vi "Test Harness.vi"() -> ()   [LabVIEW 2018]
panel:
  in  "Server Closed":string="The server VI closed the connection."
  in  "Stop":bool
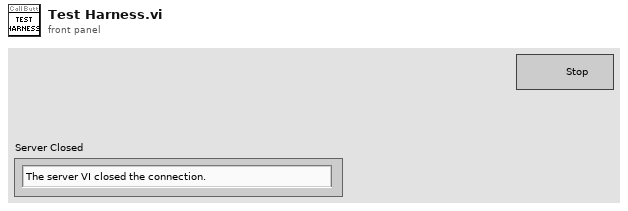
[diagram p1: front panel]
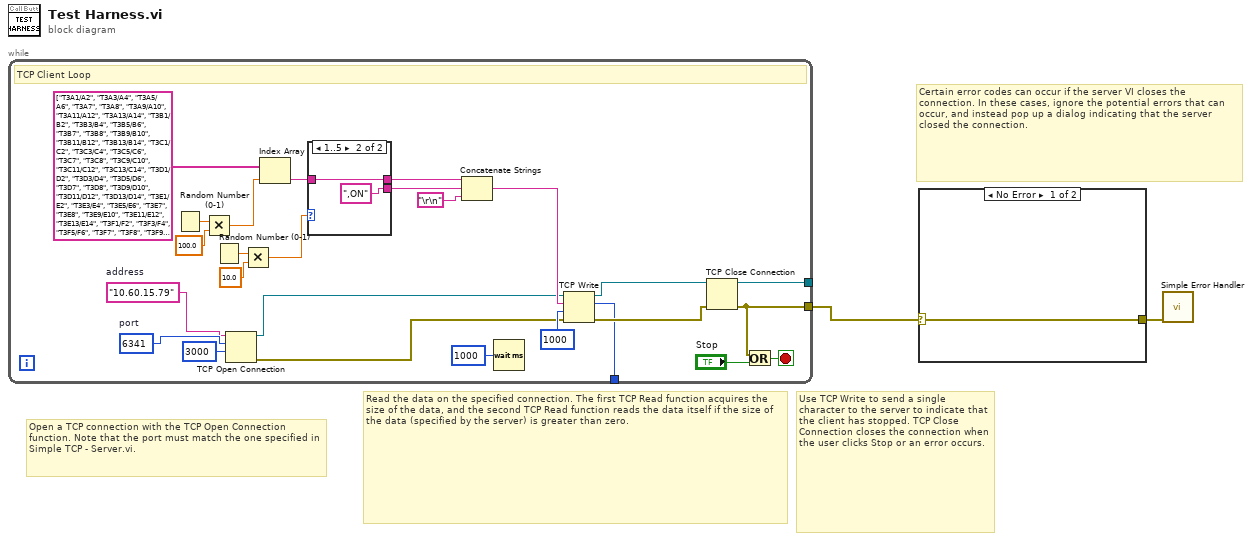
[diagram p0: block diagram]
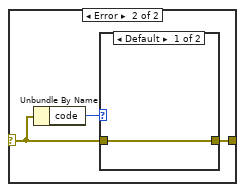
[diagram p2: hidden frame]
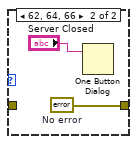
[diagram p3: hidden frame]
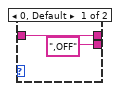
[diagram p4: hidden frame]
diagram:
  # "Certain error codes can occur if the server VI closes the connection. In these cases, ignore the potential errors that can occur, and instead pop up a dialog indicating that the server closed the connection."
  # "Use TCP Write to send a single character to the server to indicate that the client has stopped. TCP Close Connection closes the connection when the user clicks Stop or an error occurs."
  # "Read the data on the specified connection. The first TCP Read function acquires the size of the data, and the second TCP Read function reads the data itself if the size of the data (specified by the server) is greater than zero."
  # "Open a TCP connection with the TCP Open Connection function. Note that the port must match the one specified in Simple TCP - Server.vi."
  n1 = while {
    tunnel: [w10] -> w1
    tunnel: [w9] -> _
    tunnel: [w3] -> _
    stop <- w27 stop-if-true
    w7 = u16 6341  # port
    w6 = "10.60.15.79"  # address
    # "TCP Client Loop"
    n2 = Random Number (0-1)() -> (number: 0 to 1=w23:dbl)
    n3 = Multiply(x=w23, y=100.0) -> (x*y=w21:dbl)
    n4 = Random Number (0-1)() -> (number: 0 to 1=w15:dbl)
    n5 = TCP Open Connection(address=w6, remote port or service name=w7, timeout ms (60000)=3000) -> (connection ID=w5:refnum<k5>, error out=w4:errorcluster)  [unwired: 2 in]
    n6 = Multiply(x=w15, y=10.0) -> (x*y=w14:dbl)
    n7 = Index Array(array=string[] ["T3A1/A2", "T3A3/A4", "T3A5/A6", "T3A7", "T3A8", "T3A9/A10", "T3A11/A12", "T3A13/A14", "T3B1/B2", "T3B3/B4", "T3B5/B6", "T3B7", "T3B8", "T3B9/B10", "T3B11/B12", "T3B13/B14", "T3C1/C2", "T3C3/C4", "T3C5/C6", "T3C7", "T3C8", "T3C9/C10", "T3C11/C12", "T3C13/C14", "T3D1/D2", "T3D3/D4", "T3D5/D6", "T3D7", "T3D8", "T3D9/D10", "T3D11/D12", "T3D13/D14", "T3E1/E2", "T3E3/E4", "T3E5/E6", "T3E7", "T3E8", "T3E9/E10", "T3E11/E12", "T3E13/E14", "T3F1/F2", "T3F3/F4", "T3F5/F6", "T3F7", "T3F8", "T3F9/F10", "T3F11/F12", "T3F13/F14", "T3G1/G2", "T3G3/G4", "T3G5/G6", "T3G7", "T3G8", "T3G9/G10", "T3G11/G12", "T3G13/G14", "T3H1/H2", "T3H3/H4", "T3H5", "I1", "I2", "I3", "Quit", "T2B1/B2", "T2B3/B4", "T2B5/B6", "T2B7", "T2B8", "T2B9/B10", "T2B11/B12", "T2B13/B14", "T2C1/C2", "T2C3/C4", "T2C5/C6", "T2C7", "T2C8", "T2C9/C10", "T2C11/C12", "T2C13/C14", "T2D1/D2", "T2D3/D4", "T2D5/D6", "T2D7", "T2D8", "T2D9/D10", "T2D11/D12", "T2D13/D14", "T2E3/E4", "T2E5/E6", "T2E7", "T2E8", "T2E9/E10", "T2E11/E12", "T2E13/E14", "T2F1/F2", "T2F3", "T2F4/F5", "T2F6/F7", "T2G1/G2", "T2G3/G4", "T2A3/A4", "T2A5/A6", "T2A7", "T2A8", "T2A9/A10", "T2A11/A12", "T2A13/A13", "T2A1/A2", "T1B1/B2", "T1B3/B4", "T1B5/B6", "T1B7", "T1B8", "T1B9/B10", "T1B11/B12", "T1B13/B14", "T1C1/C2", "T1C3/C4", "T1C5/C6", "T1C7/C8", "T1C9/C10", "T1C11/C12", "T1D1/D2", "T1D3/D4", "T1D5/D6", "T1D7", "T1D8", "T1D9/D10", "T1D11/D12", "T1D13/D14", "T1E1/E2", "T1E3/E4", "T1E5/E6", "T1E7/E8", "T1E9/E10", "T1E11/E12", "T1F1/F2", "T1F3", "T1A3/A4", "T1A5/A6", "T1A7", "T1A8", "T1A9/A10", "T1A11/A12", "T1A13/A14", "T1A1/A2", "T2F8/F9", "T3H6/H7", "T3H8/H9", "T3H10"] ("Array"), index=w21) -> (element=w20:string)
    n8 = case shown="1..5" w14 {
      tunnel: w20 -> [w30 w32]
      tunnel: [w30 w32] -> w19
      tunnel: [",OFF" ",ON"] -> w18
      frame 0, Default {
      }
      frame 1..5 {
      }
    }
    n9 = Concatenate Strings(w19, w18, "\r\n") -> (w13:string)
    n10 = Wait (ms)(milliseconds to wait=u32 1000) -> ()  [unwired: 1 out]
    n11 = TCP Write(connection ID=w5, data in=w13, error in (no error)=w4, 9:1000 ("timeout ms (25000)")) -> (connection ID out=w11:refnum<k5>, bytes written=w3:i32, error out=w12:errorcluster)
    n12 = TCP Close Connection(connection ID=w11, error in (no error)=w12) -> (connection ID out=w9:refnum<k5>, error out=w10:errorcluster)  [unwired: 1 in]
    n13 = Or(x=w10, y="Stop") -> (x .or. y?=w27:bool)
  }
  n14 = case shown="No Error" w1 {
    selector: w1 -> [w33 w35]
    tunnel: [w33 w34] -> w2
    frame No Error {
    }
    frame Error {
      n15 = Unbundle By Name(w35) -> ("code"=w36:i32)
      n16 = case shown="Default" w36 {
        tunnel: w35 -> [w37 _]
        tunnel: [w37 w39] -> w34
        frame Default {
        }
        frame 62, 64, 66 {
          w39 = errorcluster {"status"=FALSE, "code"=0, "source"=""}  # No error
          n17 = One Button Dialog(message="Server Closed") -> ()  [unwired: 1 in, 1 out]
        }
      }
    }
  }
  n18 = call <vilib>:"Simple Error Handler.vi"("error in (no error)"=w2) -> ()  [unwired: 4 in, 5 out]
